vi "Invalid Port Error.vi"(11 "error in":errorcluster) -> (15 "error out":errorcluster)   [LabVIEW 2018]
doc: "This VI produces a standard error for an invalid port number.\n\n<B>Input Parameters</B>\n\n<B>error in</B> describes error conditions that occur before this node runs. This input provides standard error in functionality.\n\n<B>Output Parameters</B>\n\n<B>error out</B> contains error information. This output provides standard error out functionality."
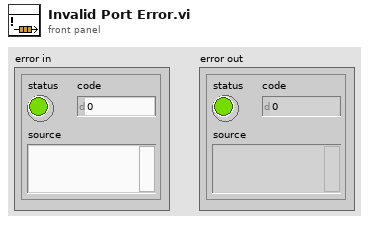
[diagram p1: front panel]
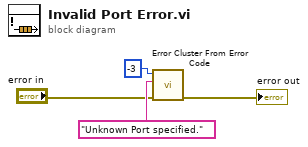
[diagram p0: block diagram]
diagram:
  n1 = call <vilib>:"Error Cluster From Error Code.vi"("error in (no error)"="error in", "error message (\"\")"="Unknown Port specified." ("error message (\"\")"), "error code (0)"=-3) -> ("error out"=→"error out":errorcluster)  [unwired: 6 in]
